vi "Lock-in sin out voltage.vi"(8 "error in (no error)":errorcluster, 9 "read-only? (t)":bool=TRUE, 10 "set voltage (V)":dbl, 11 "VISA resource name":refnum<visa-resource-name>) -> (0 "error out":errorcluster, 2 "voltage (V)":dbl, 3 "VISA resource name out":refnum<visa-resource-name>)   [LabVIEW 2009, in "Lockin SR830.lvclass"]
doc: "Sets and/or reads the current voltage of the SINE OUT output of the lock-in amplifier."
uses:
  Lockin SR830.lvclass
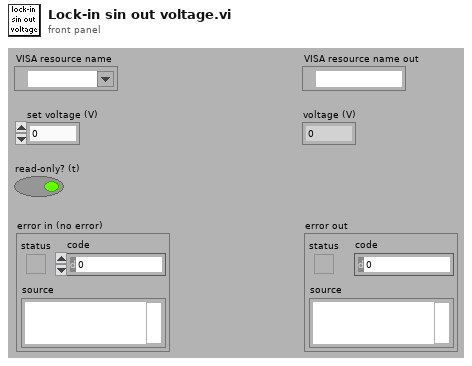
[diagram p1: front panel]
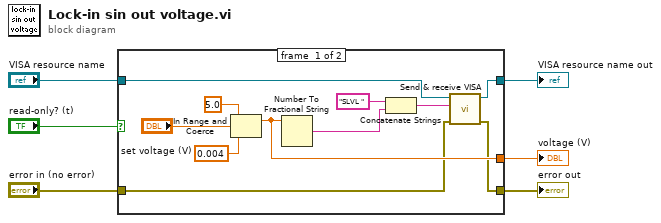
[diagram p0: block diagram]
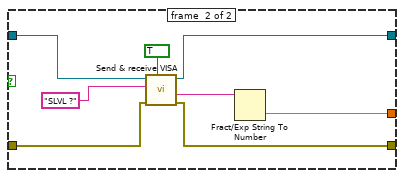
[diagram p2: hidden frame]
diagram:
  n1 = case shown="False" "read-only? (t)" {
    tunnel: [w11 w22] -> w6
    tunnel: "error in (no error)" -> [w10 w21]
    tunnel: [w9 w20] -> w3
    tunnel: "VISA resource name" -> [w8 w19]
    tunnel: [w7 w18] -> w1
    frame #0 {
      n2 = In Range and Coerce(upper limit=5.0, x="set voltage (V)", lower limit=0.004) -> (coerced(x)=w11:dbl)  [unwired: 1 out]
      n3 = Number To Fractional String(number=w11) -> (F-format string=w12:string)  [unwired: 3 out]
      n4 = Concatenate Strings("SLVL " ("write buffer"), w12) -> (w13:string)
      n5 = call "Send & receive VISA.vi"("error in (no error)"=w10, "write buffer"=w13, "VISA resource name"=w8) -> ("error out"=w9:errorcluster, "VISA resource name out"=w7:refnum<visa-resource-name>)  [unwired: 2 in, 5 out]
    }
    frame #1 {
      n6 = call "Send & receive VISA.vi"("read? (f)"=TRUE, "error in (no error)"=w21, "write buffer"="SLVL ?", "VISA resource name"=w19) -> ("error out"=w20:errorcluster, "read buffer"=w23:string, "VISA resource name out"=w18:refnum<visa-resource-name>)  [unwired: 1 in, 4 out]
      n7 = Fract/Exp String To Number(string=w23) -> (number=w22:dbl)  [unwired: 4 out]
    }
  }
  "voltage (V)" <- w6
  "error out" <- w3
  "VISA resource name out" <- w1
